vi "example_01_raw_to_calibrated.vi"() -> ()   [LabVIEW 2015, in "lv-calibration.lvlib"]
uses:
  lv-calibration.lvlib
  public/_controls/configuration.ctl
  public/_controls/type.ctl
  public/_controls/point.ctl
  public/advanced/raw_to_calibrated-scalar.vi
panel:
  in  "configuration":T1={"tag_name"="tag-123", "type"="slope_intercept", "zero"=1.0, "formula"="", "points"=[{"x"=1.0, "y"=10.0}]}
  out "value_calibrated":dbl
  out "error":errorcluster
  in  "value_raw":dbl
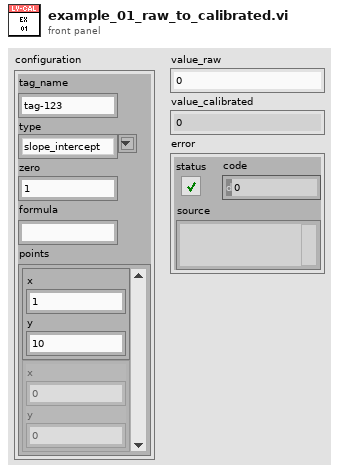
[diagram p1: front panel]
types:
  T1 = typedef "lv-calibration.lvlib/configuration.ctl" = cluster{"tag_name":string, "type":T2, "zero":dbl, "formula":string, "points":T3[]}
  T2 = typedef "lv-calibration.lvlib/type.ctl" = string
  T3 = typedef "lv-calibration.lvlib/point.ctl" = cluster{"x":dbl, "y":dbl}
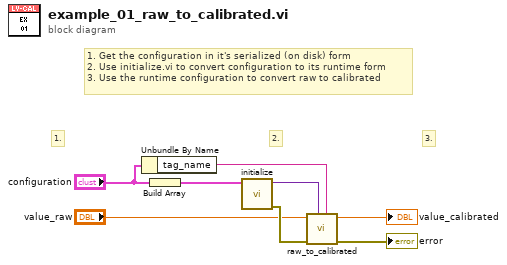
[diagram p0: block diagram]
diagram:
  # "3."
  # "2."
  # "1."
  # "1. Get the configuration in it's serialized (on disk) form\n2. Use initialize.vi to convert configuration to its runtime form\n3. Use the runtime configuration to convert raw to calibrated"
  n1 = Unbundle By Name("configuration") -> ("tag_name"=w1:string)
  n2 = Build Array("configuration") -> (w3:T1[])
  n3 = call "initialize.vi"("configuration []"=w3) -> ("error out"=w8:errorcluster, "runtime_data"=w7:variant)  [unwired: 9 in]
  n4 = call-poly "raw_to_calibrated.vi"("tag_name"=w1, "runtime"=w7, "error in (no error)"=w8, "value in"="value_raw") -> ("error out"=→"error":errorcluster, "value out"=→"value_calibrated":dbl)  [unwired: 6 in]
